vi "בדיקת מפל מתח בין הדקי הממסר תחת עומס 4.vi"(8 "error":errorcluster, 11 "Path for Log":path) -> (0 "error IO":errorcluster, 1 "בטווח כן/לא":bool, 2 "מפל מתח בין דקי הממסר תחת עומס":dbl, 3 "תוצאה זמנית":dbl)   [LabVIEW 2015]
uses:
  M9700 Driver/85/vi.lib/M9700 Modbus.llb/CTL Register Address.ctl
  M9700 Driver/86/vi.lib/M9700 Modbus.llb/CTL CMD Register.ctl
  <vilib>/DAQmx/write.llb/DAQmx Write (Digital Bool 1Line 1Point).vi
  <vilib>/Instr/_visa.llb/VISA Configure Serial Port (Instr).vi
  <vilib>/DAQmx/create/channels.llb/DAQmx Create Channel (DO-Digital Output).vi
  <vilib>/DAQmx/miscellaneous.llb/DAQmx Fill In Error Info.vi
panel:
  out "progress":dbl(slide) min=0.0 max=10.0 scale=0.0..10.0
  in  "stop":bool
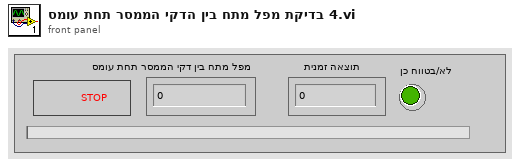
[diagram p1: front panel]
types:
  T1 = enum32{"Invalid", "Standard", "Closed", "Hidden", "Minimized", "Maximized"}
  T2 = typedef "CTL CMD Register.ctl" = u8
  T3 = typedef "CTL Register Address.ctl" = u16
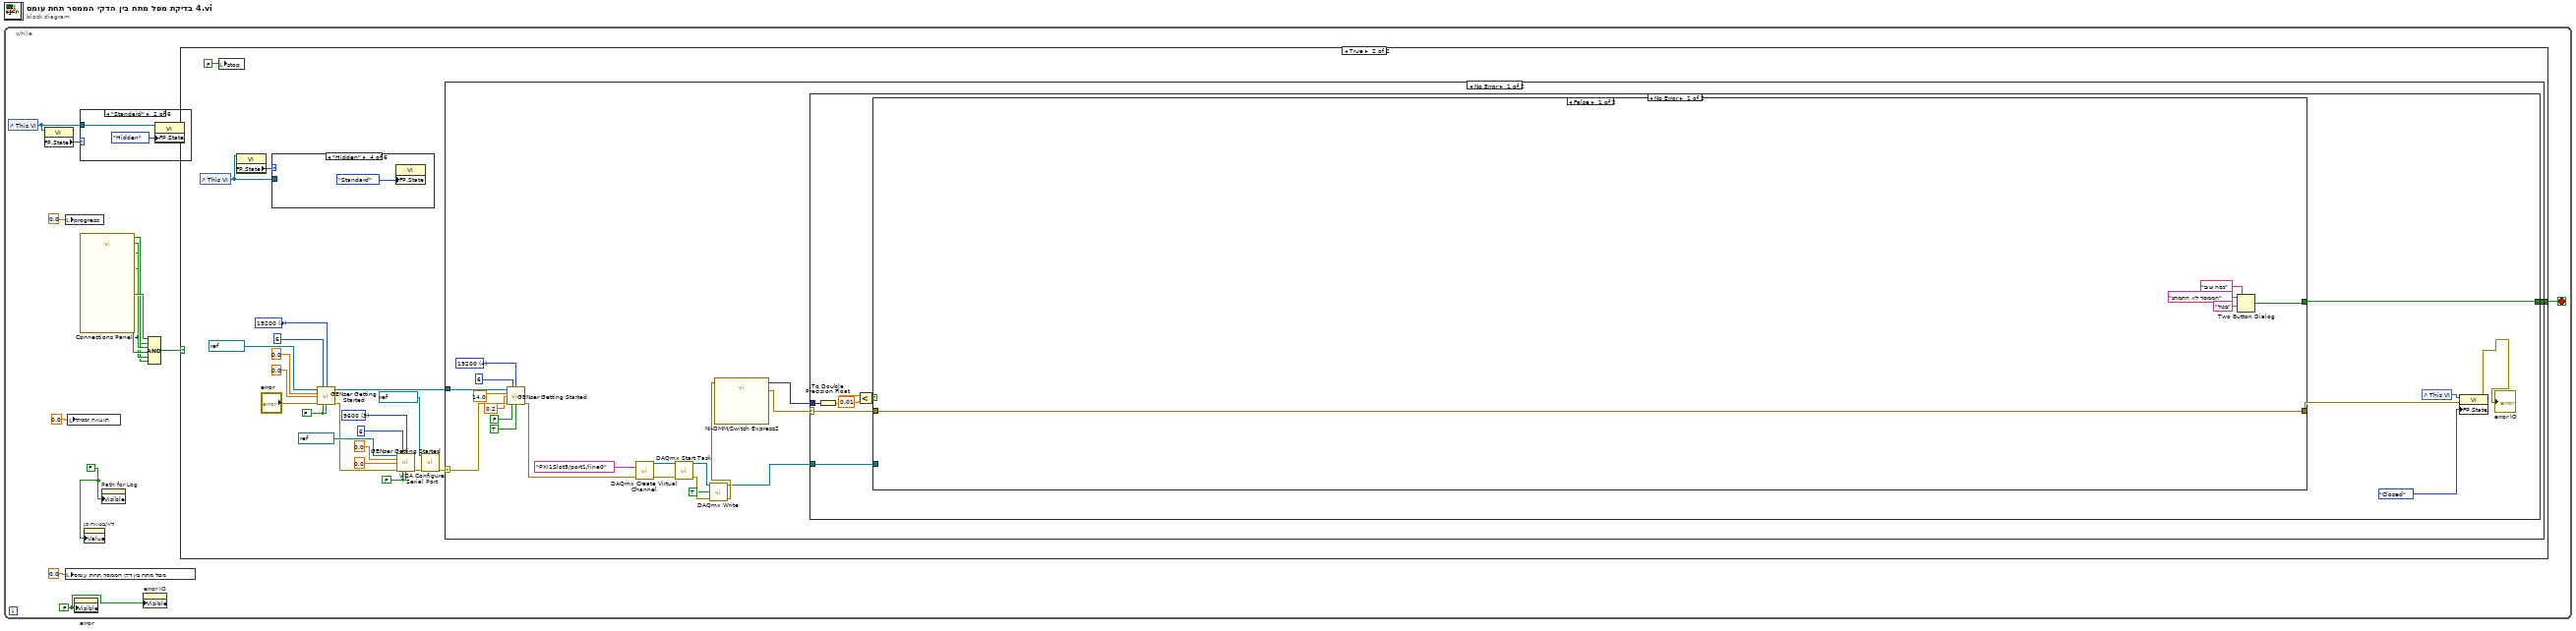
[diagram p0: block diagram]
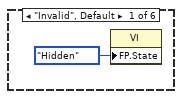
[diagram p2: hidden frame]
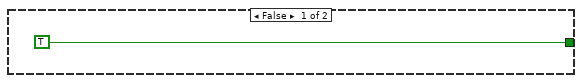
[diagram p7: hidden frame]
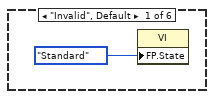
[diagram p8: hidden frame]
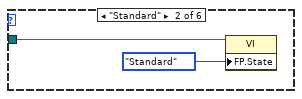
[diagram p9: hidden frame]
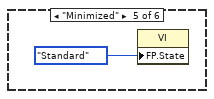
[diagram p11: hidden frame]
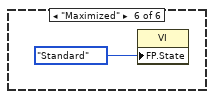
[diagram p12: hidden frame]
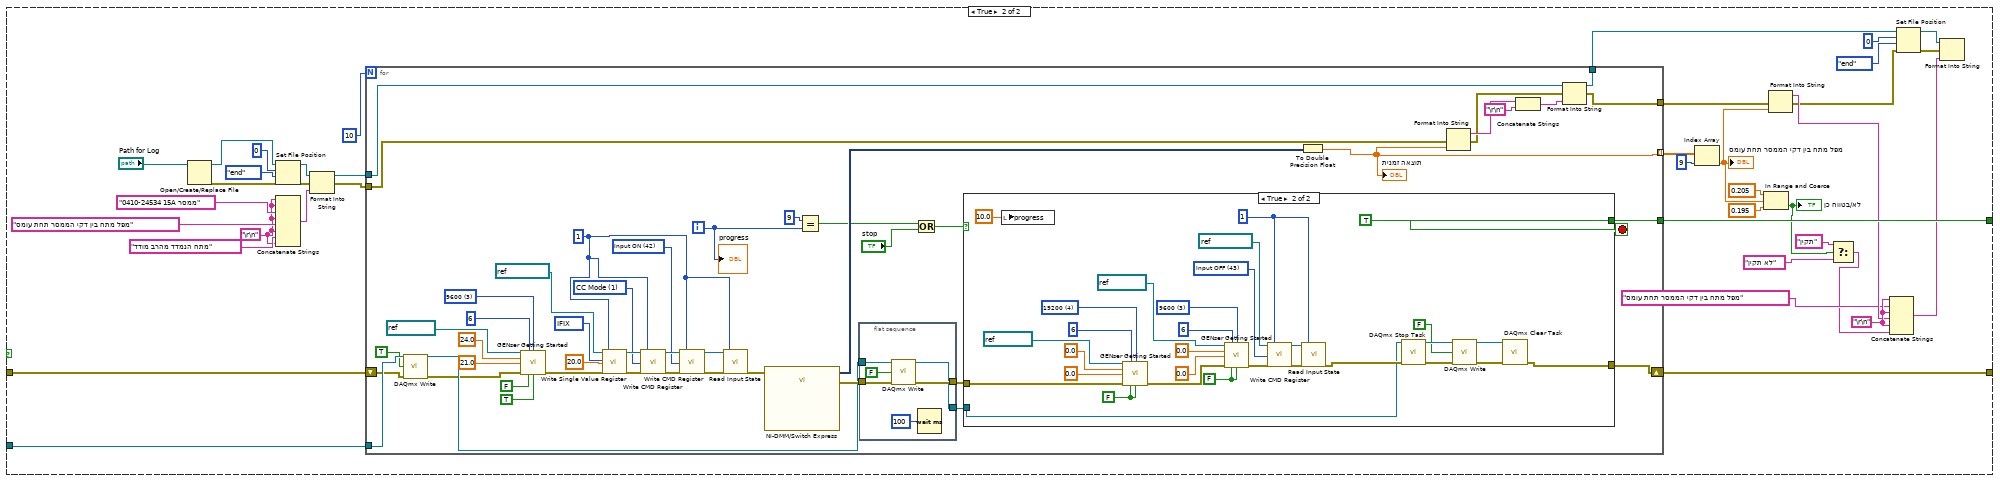
[diagram p13: hidden frame]
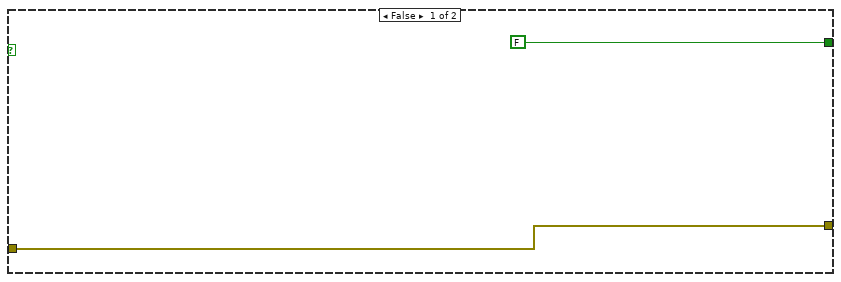
[diagram p14: hidden frame]
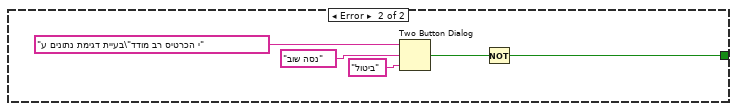
[diagram p15: hidden frame]
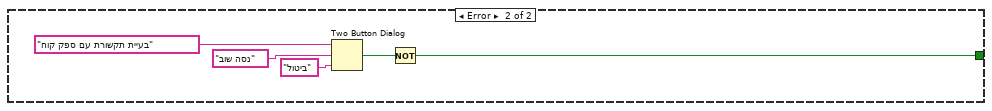
[diagram p16: hidden frame]
diagram:
  n1 = while {
    stop <- w15 stop-if-true
    w1 = FALSE ("Visible")
    w10 = FALSE ("Visible")
    n2 = control-ref of="This VI"() -> (w3:refnum<vi>)
    n3 = property class="VI"(reference=w3) -> ("FP.State"=w2:T1)  [unwired: 1 in, 2 out]
    n4 = local write "progress"(0.0 ("progress")) -> ()
    n5 = local write "מפל מתח בין דקי הממסר תחת עומס"(0.0 ("מפל מתח בין דקי הממסר תחת עומס")) -> ()
    n6 = local write "תוצאה זמנית"(0.0 ("תוצאה זמנית")) -> ()
    n7 = property on="error" class="Clust (strict)"("Visible"=w10) -> ()  [unwired: 2 in, 2 out]
    n8 = case shown="\"Standard\"" w2 {
      tunnel: w3 -> [_ w17 _ _ _ _]
      frame "Invalid", Default {
        n9 = property class="VI"("FP.State"=T1."Hidden" ("Front Panel Window:State")) -> ()  [unwired: 2 in, 2 out]
      }
      frame "Standard" {
        n10 = property class="VI"(reference=w17, "FP.State"=T1."Hidden" ("Front Panel Window:State")) -> ()  [unwired: 1 in, 2 out]
      }
      frame "Closed" {
      }
      frame "Hidden" {
      }
      frame "Minimized" {
      }
      frame "Maximized" {
      }
    }
    n11 = call "Connections Panel 4.vi"() -> ("Input Name 10"=w4:bool, "Input Name 6"=w8:bool, "Input Name 7"=w7:bool, "Input Name 8"=w6:bool, "Input Name 9"=w5:bool, "OK"=w9:bool)  [unwired: 13 in, 1 out]
    n12 = property on="בטווח כן/לא" class="Bool (strict)"("Value"=w1) -> ()  [unwired: 2 in, 2 out]
    n13 = property on="Path for Log" class="Path"("Visible"=w1) -> ()  [unwired: 2 in, 2 out]
    n14 = property on="error IO" class="Clust (strict)"("Visible"=w10) -> ()  [unwired: 2 in, 2 out]
    n15 = Compound Arithmetic op=AND(w9, w8, w7, w6, w5, w4) -> (w14:bool)
    n16 = case shown="True" w14 {
      tunnel: [TRUE w28] -> w15
      frame False {
      }
      frame True {
        w24 = FALSE ("Reset (T)")
        w33 = u16 3 items=["1200", "2400", "4800", "9600", "19200"] ("BAUD")
        w23 = FALSE ("Output On (T)")
        w38 = u16 4 items=["1200", "2400", "4800", "9600", "19200"] ("BAUD")
        n17 = control-ref of="This VI"() -> (w20:refnum<vi>)
        n18 = local write "stop"(FALSE ("stop")) -> ()
        n19 = property class="VI"(reference=w20) -> ("FP.State"=w21:T1)  [unwired: 1 in, 2 out]
        n20 = case shown="\"Hidden\"" w21 {
          tunnel: w20 -> [_ w43 _ _ _ _]
          frame "Invalid", Default {
            n21 = property class="VI"("FP.State"=T1."Standard" ("Front Panel Window:State")) -> ()  [unwired: 2 in, 2 out]
          }
          frame "Standard" {
            n22 = property class="VI"(reference=w43, "FP.State"=T1."Standard" ("Front Panel Window:State")) -> ()  [unwired: 1 in, 2 out]
          }
          frame "Closed" {
          }
          frame "Hidden" {
            n23 = property class="VI"("FP.State"=T1."Standard" ("Front Panel Window:State")) -> ()  [unwired: 2 in, 2 out]
          }
          frame "Minimized" {
            n24 = property class="VI"("FP.State"=T1."Standard" ("Front Panel Window:State")) -> ()  [unwired: 2 in, 2 out]
          }
          frame "Maximized" {
            n25 = property class="VI"("FP.State"=T1."Standard" ("Front Panel Window:State")) -> ()  [unwired: 2 in, 2 out]
          }
        }
        n26 = call "GENser Getting Started.vi"("VISA"=refnum<visa-resource-name> "COM6", "GEN Addr"=i16 6, "BAUD"=w38, "Voltage Limit"=0.0, "Current Limit"=0.0, "error"="error", "Reset (T)"=w23, "Output On (T)"=w23) -> ("VISA out"=w40:refnum<visa-resource-name>, "error out"=w29:errorcluster)  [unwired: 4 in, 2 out]
        n27 = call "GENser Getting Started.vi"("VISA"=refnum<visa-resource-name> "COM4", "GEN Addr"=i16 6, "BAUD"=w33, "Voltage Limit"=0.0, "Current Limit"=0.0, "error"=w29, "Reset (T)"=w24, "Output On (T)"=w24) -> ("error out"=w26:errorcluster)  [unwired: 4 in, 3 out]
        n28 = call-poly "VISA Configure Serial Port"("VISA resource name"=refnum<visa-resource-name> "COM13", "error in (no error)"=w26) -> ("error out"=w25:errorcluster)  [unwired: 4 in, 9 out]
        n29 = case shown="No Error" w25 {
          selector: w25 -> [w64 _]
          tunnel: w40 -> [w67 _]
          tunnel: [w66 w212] -> w28
          frame No Error {
            w58 = u16 4 items=["1200", "2400", "4800", "9600", "19200"] ("BAUD")
            n30 = call "GENser Getting Started.vi"("VISA"=w67, "GEN Addr"=i16 6, "BAUD"=w58, "Voltage Limit"=14.0, "Current Limit"=0.2, "error"=w64, "Reset (T)"=FALSE, "Output On (T)"=TRUE) -> ("error out"=w50:errorcluster)  [unwired: 4 in, 3 out]
            n31 = call-poly <vilib>:"DAQmx Create Virtual Channel.vi"("lines"=tag "PXI1Slot5/port1/line0", "error in"=w50) -> ("task out"=w56:refnum<k21>, "error out"=w57:errorcluster)  [unwired: 12 in]
            n32 = call <vilib>:"DAQmx Start Task.vi"("task/channels in"=w56, "error in"=w57) -> ("task out"=w49:refnum<k21>, "error out"=w52:errorcluster)  [unwired: 12 in]
            n33 = call-poly <vilib>:"DAQmx Write.vi"("task/channels in"=w49, "data"=TRUE, "error in"=w52) -> ("task out"=w48:refnum<k21>, "error out"=w53:errorcluster)  [unwired: 10 in, 1 out]
            n34 = call "NI-DMM/Switch Express2"("error in"=w53) -> ("signals out"=w65:dynamicdata, "error out"=w54:errorcluster)  [unwired: 16 in, 1 out]
            n35 = case shown="No Error" w54 {
              selector: w54 -> [w76 _]
              tunnel: [w75 w207] -> w66
              tunnel: w65 -> [w78 _]
              tunnel: w48 -> [w69 _]
              frame No Error {
                n36 = To Double Precision Float(number=w78) -> (double precision float=w74:dbl)
                n37 = Less?(x=w74, y=0.01) -> (x < y?=w77:bool)
                n38 = case shown="False" w77 {
                  tunnel: w76 -> [w83 w120]
                  tunnel: [w82 w121] -> w75
                  tunnel: [w83 w114] -> w70
                  tunnel: w69 -> [_ w115]
                  frame False {
                    n39 = Two Button Dialog(message="הממסר לא התמתג", 1:"נסה שוב" ("F button name (\"Cancel\")"), 2:"בטל" ("T button name (\"OK\")")) -> (T button?=w82:bool)
                  }
                  frame True {
                    w99 = "\r\n"
                    w102 = "\r\n"
                    n40 = Open/Create/Replace File(file path (use dialog)="Path for Log") -> (refnum out=w111:refnum<file>, error out=w110:errorcluster)  [unwired: 5 in, 1 out]
                    n41 = Set File Position(offset (in bytes) (0)=i64 0, refnum=w111, from (0:start)=enum16{"start", "end", "current"}."end", error in=w110) -> (refnum out=w106:refnum<file>, error out=w103:errorcluster)
                    n42 = Concatenate Strings(w102, w102, "0410-24534 15A ממסר", w102, "מפל מתח בין דקי הממסר תחת עומס", w102, "מתח הנמדד מהרב מודד", w102) -> (w109:string)
                    n43 = Format Into String(initial string=w106, error in=w103, w109) -> (resulting string=w100:refnum<file>, error out=w101:errorcluster)  [unwired: 1 in]
                    n44 = for {
                      N: 10 -> [_]
                      tunnel: [w144] -> w121
                      shift-right: [w141] -> w114
                      shift-left: w120 -> [w136]
                      tunnel: [w123] -> w119 mode=indexing
                      tunnel: w115 -> [w137]
                      tunnel: w101 -> [w126]
                      tunnel: w100 -> [w128]
                      tunnel: [w125] -> w93
                      tunnel: [w124] -> w84
                      i -> [w140]
                      stop <- w144 stop-if-true
                      w152 = T2 42 items=["CC Mode"=1, "CV Mode"=2, "CW Mode"=3, "CR Mode"=4, "Short Mode"=26, "Set SysPara"=41, "Input ON"=42, "Input OFF"=43] ("CMD Register Value")
                      w155 = u8 1 ("Load Address")
                      w159 = T2 1 items=["CC Mode"=1, "CV Mode"=2, "CW Mode"=3, "CR Mode"=4, "Short Mode"=26, "Set SysPara"=41, "Input ON"=42, "Input OFF"=43] ("CMD Register Value")
                      w162 = T3 2561 items=["REMOTE"=1283, "ISTATE"=1296, "CMD"=2560, "IFIX"=2561, "UFIX"=2563, "PFIX"=2565, "RFIX"=2567, "IMAX"=2612, "UMAX"=2614, "PMAX"=2616, "U"=2816, "I"=2818, "MODEL"=2822, "EDITION"=2823] ("Register Address")
                      w167 = u16 3 items=["1200", "2400", "4800", "9600", "19200"] ("BAUD")
                      n45 = call-poly <vilib>:"DAQmx Write.vi"("task/channels in"=w137, "data"=TRUE, "error in"=w136) -> ("task out"=w135:refnum<k21>, "error out"=w134:errorcluster)  [unwired: 10 in, 1 out]
                      n46 = call "GENser Getting Started.vi"("VISA"=refnum<visa-resource-name> "COM4", "GEN Addr"=i16 6, "BAUD"=w167, "Voltage Limit"=24.0, "Current Limit"=21.0, "error"=w134, "Reset (T)"=FALSE, "Output On (T)"=TRUE) -> ("error out"=w157:errorcluster)  [unwired: 4 in, 3 out]
                      n47 = call "Write Single Value Register.vi"("VISA resource name"=refnum<visa-resource-name> "COM13", "Starting Address(HEX)"=w162, "Register Single Value"=sgl 20.0, "error in"=w157, "Load Address"=w155) -> ("VISA resource name out"=w161:refnum<visa-resource-name>, "error out"=w160:errorcluster)  [unwired: 13 out]
                      n48 = call "Write CMD Register.vi"("VISA resource name"=w161, "CMD Value"=w159, "error in"=w160, "Load Address"=w155) -> ("VISA resource name out"=w156:refnum<visa-resource-name>, "error out"=w153:errorcluster)  [unwired: 14 out]
                      n49 = call "Write CMD Register.vi"("VISA resource name"=w156, "CMD Value"=w152, "error in"=w153, "Load Address"=w155) -> ("VISA resource name out"=w154:refnum<visa-resource-name>, "error out"=w151:errorcluster)  [unwired: 14 out]
                      n50 = call "Read Input State.vi"("VISA resource name"=w154, "error in"=w151, "Load Address"=w155) -> ("error out"=w150:errorcluster)  [unwired: 16 out]
                      n51 = call "NI-DMM/Switch Express"("error in"=w150) -> ("signals out"=w149:dynamicdata, "error out"=w138:errorcluster)  [unwired: 16 in, 1 out]
                      n52 = Equal?(x=9, y=w140) -> (x = y?=w146:bool)
                      n53 = flat-sequence {
                        tunnel: [w174] -> w139
                        tunnel: w138 -> [w173]
                        tunnel: w135 -> [w171]
                        tunnel: [w170] -> w132
                        frame #0 {
                          n54 = call-poly <vilib>:"DAQmx Write.vi"("task/channels in"=w171, "data"=FALSE, "error in"=w173) -> ("task out"=w170:refnum<k21>, "error out"=w174:errorcluster)  [unwired: 10 in, 1 out]
                          n55 = Wait (ms)(milliseconds to wait=u32 100) -> ()  [unwired: 1 out]
                        }
                      }
                      n56 = Or(x=w146, y="stop") -> (x .or. y?=w147:bool)
                      n57 = case shown="True" w147 {
                        tunnel: [FALSE TRUE] -> w144
                        tunnel: w139 -> [w175 w195]
                        tunnel: [w175 w178] -> w141
                        tunnel: w132 -> [_ w177]
                        frame False {
                        }
                        frame True {
                          w186 = u8 1 ("Load Address")
                          w189 = T2 43 items=["CC Mode"=1, "CV Mode"=2, "CW Mode"=3, "CR Mode"=4, "Short Mode"=26, "Set SysPara"=41, "Input ON"=42, "Input OFF"=43] ("CMD Register Value")
                          w193 = FALSE ("Reset (T)")
                          w199 = u16 3 items=["1200", "2400", "4800", "9600", "19200"] ("BAUD")
                          w192 = FALSE ("Reset (T)")
                          w202 = u16 4 items=["1200", "2400", "4800", "9600", "19200"] ("BAUD")
                          n58 = local write "progress"(10.0 ("progress")) -> ()
                          n59 = call "GENser Getting Started.vi"("VISA"=refnum<visa-resource-name> "COM6", "GEN Addr"=i16 6, "BAUD"=w202, "Voltage Limit"=0.0, "Current Limit"=0.0, "error"=w195, "Reset (T)"=w192, "Output On (T)"=w192) -> ("error out"=w194:errorcluster)  [unwired: 4 in, 3 out]
                          n60 = call "GENser Getting Started.vi"("VISA"=refnum<visa-resource-name> "COM4", "GEN Addr"=i16 6, "BAUD"=w199, "Voltage Limit"=0.0, "Current Limit"=0.0, "error"=w194, "Reset (T)"=w193, "Output On (T)"=w193) -> ("error out"=w191:errorcluster)  [unwired: 4 in, 3 out]
                          n61 = call "Write CMD Register.vi"("VISA resource name"=refnum<visa-resource-name> "COM13", "CMD Value"=w189, "error in"=w191, "Load Address"=w186) -> ("VISA resource name out"=w187:refnum<visa-resource-name>, "error out"=w190:errorcluster)  [unwired: 14 out]
                          n62 = call "Read Input State.vi"("VISA resource name"=w187, "error in"=w190, "Load Address"=w186) -> ("error out"=w179:errorcluster)  [unwired: 16 out]
                          n63 = call <vilib>:"DAQmx Stop Task.vi"("task/channels in"=w177, "error in"=w179) -> ("task out"=w184:refnum<k21>, "error out"=w182:errorcluster)  [unwired: 12 in]
                          n64 = call-poly <vilib>:"DAQmx Write.vi"("task/channels in"=w184, "data"=FALSE, "error in"=w182) -> ("task out"=w181:refnum<k21>, "error out"=w180:errorcluster)  [unwired: 10 in, 1 out]
                          n65 = call <vilib>:"DAQmx Clear Task.vi"("task in"=w181, "error in"=w180) -> ("error out"=w178:errorcluster)  [unwired: 13 in]
                        }
                      }
                      n66 = To Double Precision Float(number=w149) -> (double precision float=w123:dbl)
                      "תוצאה זמנית" <- w123
                      n67 = Format Into String(error in=w126, w123) -> (resulting string=w130:string, error out=w127:errorcluster)  [unwired: 2 in]
                      n68 = Concatenate Strings(w130, "\r\n") -> (w129:string)
                      n69 = Format Into String(initial string=w128, error in=w127, w129) -> (resulting string=w125:refnum<file>, error out=w124:errorcluster)  [unwired: 1 in]
                      "progress" <- w140
                    }
                    n70 = Index Array(array=w119, index=9) -> (element=w92:dbl)
                    "מפל מתח בין דקי הממסר תחת עומס" <- w92
                    n71 = In Range and Coerce(upper limit=0.205, x=w92, lower limit=0.195) -> (In Range?=w87:bool)  [unwired: 1 out]
                    "בטווח כן/לא" <- w87
                    n72 = Format Into String(error in=w84, w92) -> (resulting string=w91:string, error out=w85:errorcluster)  [unwired: 2 in]
                    n73 = Select(t="תקין", s=w87, f="לא תקין") -> (s? t:f=w86:string)
                    n74 = Concatenate Strings(w99, "מפל מתח בין דקי הממסר תחת עומס" ("string"), w99, w91, w99, w86) -> (w94:string)
                    n75 = Set File Position(offset (in bytes) (0)=i64 0, refnum=w93, from (0:start)=enum16{"start", "end", "current"}."end", error in=w85) -> (refnum out=w96:refnum<file>, error out=w95:errorcluster)
                    n76 = Format Into String(initial string=w96, error in=w95, w94) -> ()  [unwired: 1 in, 2 out]
                  }
                }
                n77 = control-ref of="This VI"() -> (w72:refnum<vi>)
                n78 = property class="VI"(reference=w72, error in=w70, "FP.State"=T1."Closed" ("Front Panel Window:State")) -> (error out=→"error IO":errorcluster)  [unwired: 1 out]
              }
              frame Error {
                n79 = Two Button Dialog(message="בעיית דגימת נתונים ע\"י הכרטיס רב מודד", 1:"ביטול" ("F button name (\"Cancel\")"), 2:"נסה שוב" ("T button name (\"OK\")")) -> (T button?=w208:bool)
                n80 = Not(x=w208) -> (.not. x?=w207:bool)
              }
            }
          }
          frame Error {
            n81 = Two Button Dialog(message="בעיית תקשורת עם ספק קוח", 1:"ביטול" ("F button name (\"Cancel\")"), 2:"נסה שוב" ("T button name (\"OK\")")) -> (T button?=w213:bool)
            n82 = Not(x=w213) -> (.not. x?=w212:bool)
          }
        }
      }
    }
  }
